vi "MKS CTLR - Read Serial Data.vi"(6 "Read timeout (mSec)":u64=10, 8 "error in (no error)":errorcluster, 11 "VISA resource name (IN)":refnum<visa-resource-name>) -> (0 "error out":errorcluster, 3 "VISA resource name (OUT)":refnum<visa-resource-name>, 5 "Response":string)   [LabVIEW 2013]
panel:
  out "Bytes at Port":u32
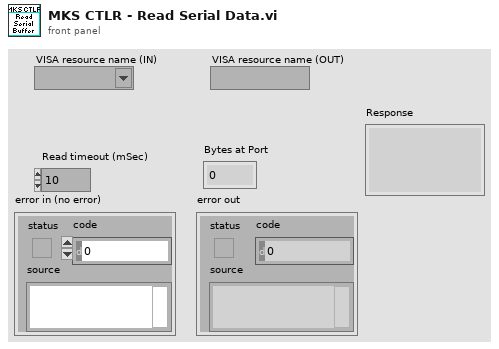
[diagram p1: front panel]
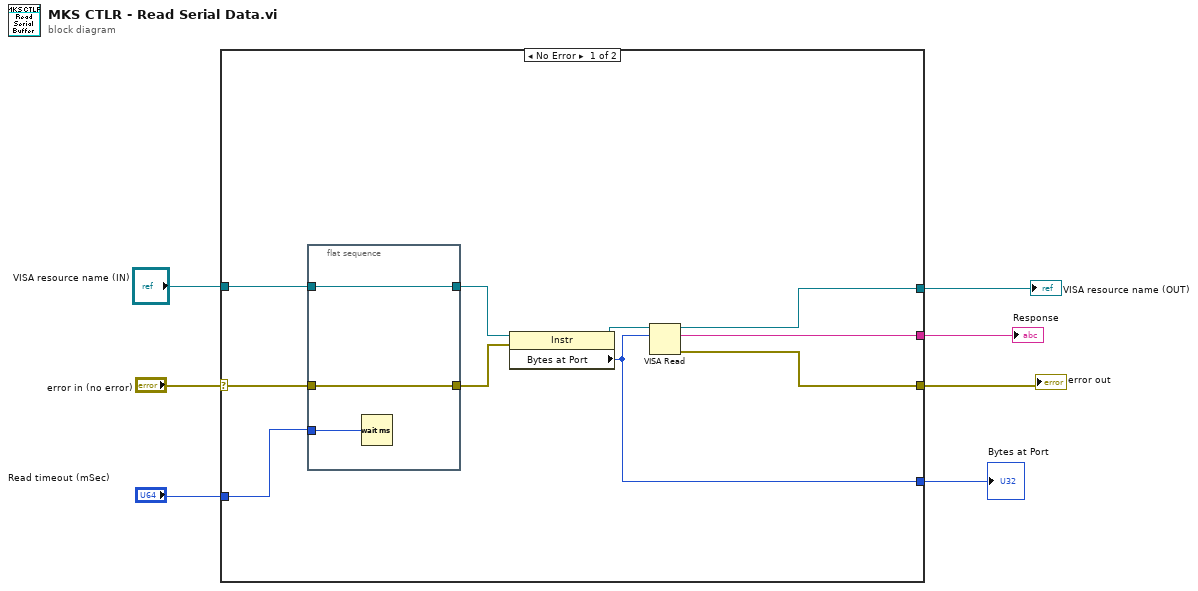
[diagram p0: block diagram]
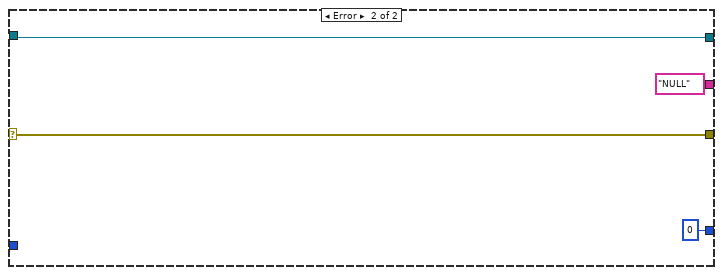
[diagram p2: hidden frame]
diagram:
  n1 = case shown="No Error" "error in (no error)" {
    selector: "error in (no error)" -> [w16 w23]
    tunnel: "VISA resource name (IN)" -> [w15 w24]
    tunnel: "Read timeout (mSec)" -> [w17 _]
    tunnel: [w12 u32 0 ("Bytes at Port")] -> w4
    tunnel: [w11 w23] -> w3
    tunnel: [w10 w24] -> w2
    tunnel: [w9 "NULL" ("read buffer")] -> w1
    frame No Error {
      n2 = flat-sequence {
        tunnel: w17 -> [w20]
        tunnel: w16 -> [w19]
        tunnel: [w19] -> w14
        tunnel: w15 -> [w18]
        tunnel: [w18] -> w13
        frame #0 {
          n3 = Wait (ms)(milliseconds to wait=w20) -> ()  [unwired: 1 out]
        }
      }
      n4 = property class="Instr"(reference=w13, error in=w14) -> (reference out=w8:refnum<visa-resource-name>, "Bytes at Port"=w12:u32)  [unwired: 1 out]
      n5 = VISA Read(VISA resource name=w8, byte count=w12) -> (VISA resource name out=w10:refnum<visa-resource-name>, read buffer=w9:string, error out=w11:errorcluster)  [unwired: 1 in, 1 out]
    }
    frame Error {
    }
  }
  "error out" <- w3
  "VISA resource name (OUT)" <- w2
  "Bytes at Port" <- w4
  "Response" <- w1
